vi "ChassisSpeeds_FromFieldRelativeSpeeds.vi"(8 "RobotAngle":T1={"VALUE"=0.0, "COS"=1.0, "SIN"=0.0} {"SIN" format="%13.4f"; "COS" format="%13.4f"; "VALUE" format="%13.4f"}, 9 "Omega":dbl, 10 "vY":dbl, 11 "vX":dbl) -> (3 "CHASSIS":T2 {"vOmega" format="%10.3f"; "vY" format="%10.3f"; "vX" format="%10.3f"})   [LabVIEW 2019, in "Trajectory_Library.lvlib"]
doc: "Converts a user provided field-relative set of speeds into a robot-relative ChassisSpeeds object.\n\nParameters: \n - VX - The component of speed in the x direction relative to the field. Positive x is away from your alliance wall. (Meters/sec)\n - VY - The component of speed in the y direction relative to the field. Positive y is to your left when standing behind the alliance wall. (Meters/sec)\n -omega - The angular rate of the robot. (Radians/Sec)\n -robotAngle - The angle of the robot as measured by a gyroscope. The robot's angle is considered to be zero when it is facing directly away from your alliance station wall. Remember that this should be CCW positive. (radians)\n\nReturns:\n - ChassisSpeeds - Data structure representing the speeds in the robot's frame of reference."
uses:
  Trajectory_Library.lvlib
  CHASSIS_SPEEDS.ctl
  ROTATION2D.ctl
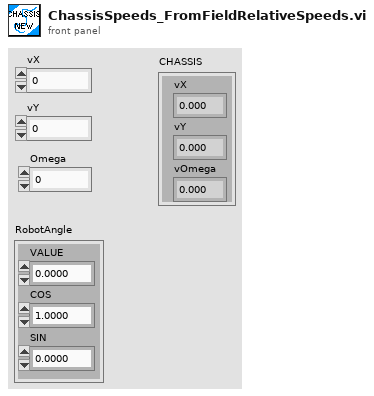
[diagram p1: front panel]
types:
  T1 = typedef "Trajectory_Library.lvlib/ROTATION2D.ctl" = cluster{"VALUE":dbl, "COS":dbl, "SIN":dbl}
  T2 = typedef "Trajectory_Library.lvlib/CHASSIS_SPEEDS.ctl" = cluster{"vX":dbl, "vY":dbl, "vOmega":dbl}
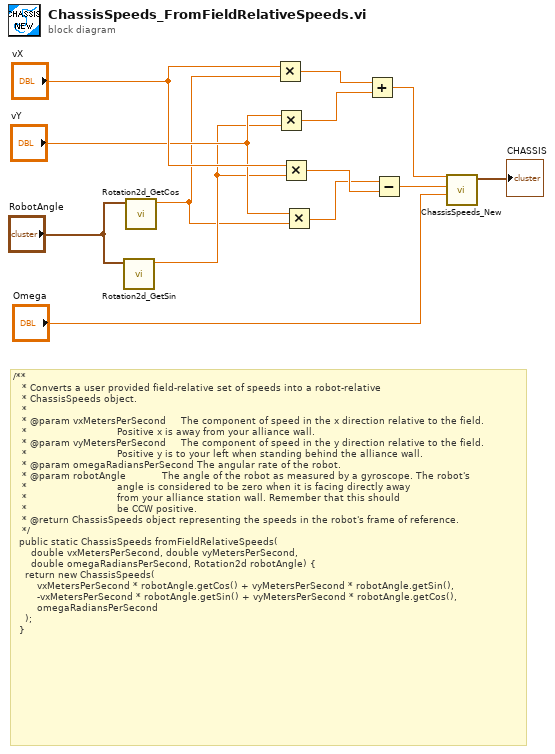
[diagram p0: block diagram]
diagram:
  # "/**\n   * Converts a user provided field-relative set of speeds into a robot-relative\n   * ChassisSpeeds object.\n   *\n   * @param vxMetersPerSecond     The component of speed in the x direction relative to the field.\n   *                              Positive x is away from your alliance wall.\n   * @param vyMetersPerSecond     The component of speed in the y direction relative to the field.\n   *                              Positive y is to your left when standing behind the alliance wall.\n   * @param omegaRadiansPerSecond The angular rate of the robot.\n   * @param robotAngle            The angle of the robot as measured by a gyroscope. The robot's\n   *                              angle is considered to be zero when it is facing directly away\n   *                              from your alliance station wall. Remember that this should\n   *                              be CCW positive.\n   * @return ChassisSpeeds object representing the speeds in the robot's frame of reference.\n   */\n  public static ChassisSpeeds fromFieldRelativeSpeeds(\n      double vxMetersPerSecond, double vyMetersPerSecond,\n      double omegaRadiansPerSecond, Rotation2d robotAngle) {\n    return new ChassisSpeeds(\n        vxMetersPerSecond * robotAngle.getCos() + vyMetersPerSecond * robotAngle.getSin(),\n        -vxMetersPerSecond * robotAngle.getSin() + vyMetersPerSecond * robotAngle.getCos(),\n        omegaRadiansPerSecond\n    );\n  }"
  n1 = call "Rotation2d_GetSin.vi"("in ROTATION"="RobotAngle") -> ("SINE"=w2:dbl)  [unwired: 10 in]
  n2 = call "Rotation2d_GetCos.vi"("in ROTATION"="RobotAngle") -> ("Cos"=w1:dbl)  [unwired: 10 in]
  n3 = Multiply(x="vX", y=w1) -> (x*y=w9:dbl)
  n4 = Multiply(x="vY", y=w2) -> (x*y=w8:dbl)
  n5 = Multiply(x="vX", y=w2) -> (x*y=w7:dbl)
  n6 = Multiply(x="vY", y=w1) -> (x*y=w6:dbl)
  n7 = Add(x=w9, y=w8) -> (x+y=w5:dbl)
  n8 = Subtract(x=w6, y=w7) -> (x-y=w4:dbl)
  n9 = call "ChassisSpeeds_New.vi"("vAngular"="Omega", "vY"=w4, "vX"=w5) -> ("CHASSIS"=→"CHASSIS":T2)  [unwired: 8 in]
